vi "Initialize.vi"(8 "error in (no error)":errorcluster, 11 "Stage_MadCityLab in":refnum<class "Stage_MadCityLab.lvclass">) -> (0 "error out":errorcluster, 3 "Stage_MadCityLab out":refnum<class "Stage_MadCityLab.lvclass">)   [LabVIEW 2020, in "Stage_MadCityLab.lvlib" / "Stage_MadCityLab.lvclass"]
uses:
  Stage_MadCityLab.lvclass
  Stage_MadCityLab.lvclass/Stage_MadCityLab.ctl
  HAL Layer/Stage/Stage/Stage.lvclass
  Dependency/Madlib.dll
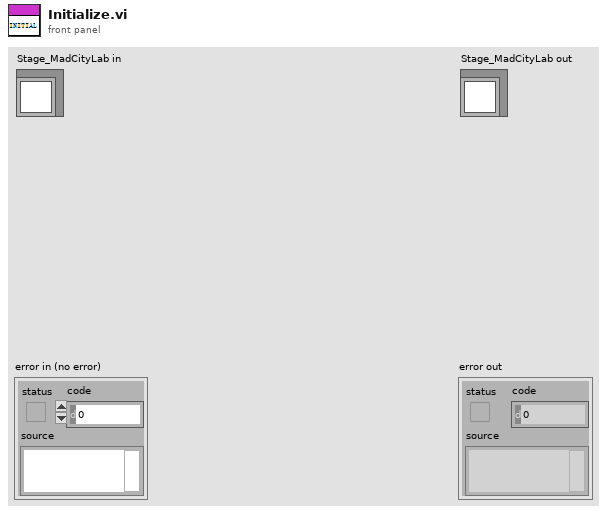
[diagram p1: front panel]
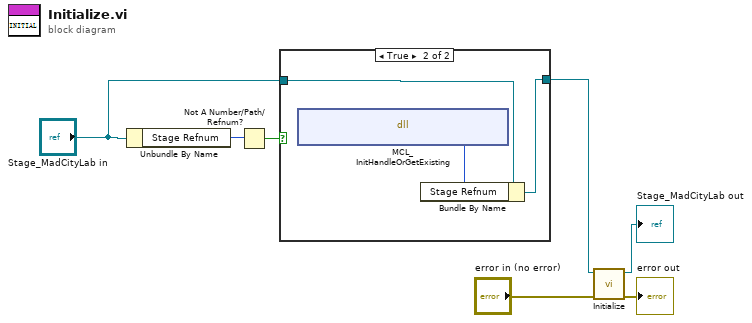
[diagram p0: block diagram]
diagram:
  n1 = Unbundle By Name("Stage_MadCityLab in") -> ("Stage Refnum"=w4:i32)
  n2 = Not A Number/Path/Refnum?(number/path/refnum=w4) -> (NaN/Path/Refnum?=w3:bool)
  n3 = case shown="True" w3 {
    tunnel: "Stage_MadCityLab in" -> [w8 w10]
    tunnel: [w8 w9] -> w1
    frame False {
    }
    frame True {
      n4 = dll-call lib="E:/Development/DevHardSoftware/MMicroscopyAF/Model/Real Hardware/Stage_MadCityLab/Stage_MadCityLab/Dependency/Madlib.dll" fn="MCL_InitHandleOrGetExisting"() -> ("return type"=w11:i32)  [unwired: 3 in, 2 out]
      n5 = Bundle By Name(cluster=w10, "Stage Refnum"=w11) -> (w9:refnum<class "Stage_MadCityLab.lvclass">)
    }
  }
  n6 = call-parent "Initialize.vi"("error in (no error)"="error in (no error)", "Device in"=w1) -> ("error out"=→"error out":errorcluster, "Device out"=→"Stage_MadCityLab out":refnum<class "Stage_MadCityLab.lvclass">)  [unwired: 8 in]
